vi "#24_MAV_MSG_GPS_RAW_INT.vi"(11 "mavlink_payload":u8[](array[numeric])) -> (3 "GPS_RAW_INT":T1)   [LabVIEW 2023]
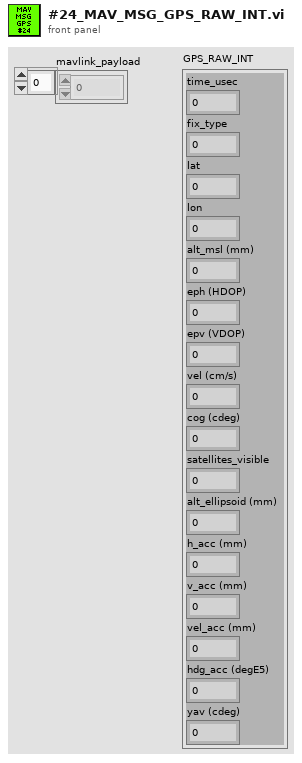
[diagram p1: front panel]
types:
  T1 = cluster{"time_usec":u64, "fix_type":u8, "lat":i32, "lon":i32, "alt_msl (mm)":i32, "eph (HDOP)":u16, "epv (VDOP)":u16, "vel (cm/s)":u16, "cog (cdeg)":u16, "satellites_visible":u8, "alt_ellipsoid (mm)":i32, "h_acc (mm)":u32, "v_acc (mm)":u32, "vel_acc (mm)":u32, "hdg_acc (degE5)":u32, "yav (cdeg)":u16}
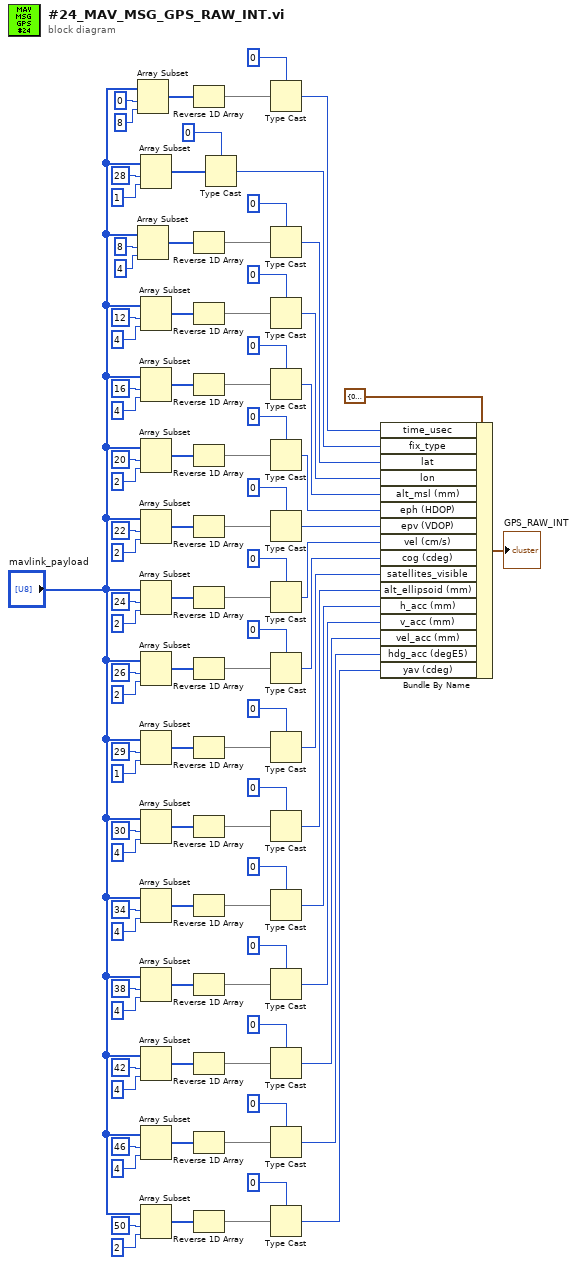
[diagram p0: block diagram]
diagram:
  n1 = Array Subset(array="mavlink_payload", index=0, length=8) -> (w98:u8[])
  n2 = Array Subset(array="mavlink_payload", index=8, length=4) -> (w82:u8[])
  n3 = Array Subset(array="mavlink_payload", index=28, length=1) -> (w88:u8[])
  n4 = Array Subset(array="mavlink_payload", index=12, length=4) -> (w76:u8[])
  n5 = Array Subset(array="mavlink_payload", index=16, length=4) -> (w70:u8[])
  n6 = Array Subset(array="mavlink_payload", index=20, length=2) -> (w65:u8[])
  n7 = Array Subset(array="mavlink_payload", index=22, length=2) -> (w59:u8[])
  n8 = Array Subset(array="mavlink_payload", index=24, length=2) -> (w53:u8[])
  n9 = Array Subset(array="mavlink_payload", index=26, length=2) -> (w47:u8[])
  n10 = Array Subset(array="mavlink_payload", index=29, length=1) -> (w41:u8[])
  n11 = Array Subset(array="mavlink_payload", index=30, length=4) -> (w35:u8[])
  n12 = Array Subset(array="mavlink_payload", index=34, length=4) -> (w29:u8[])
  n13 = Array Subset(array="mavlink_payload", index=38, length=4) -> (w23:u8[])
  n14 = Array Subset(array="mavlink_payload", index=42, length=4) -> (w17:u8[])
  n15 = Array Subset(array="mavlink_payload", index=46, length=4) -> (w11:u8[])
  n16 = Array Subset(array="mavlink_payload", index=50, length=2) -> (w5:u8[])
  n17 = Reverse 1D Array(array=w98) -> (reversed array=w97:u8[])
  n18 = Reverse 1D Array(array=w82) -> (reversed array=w81:u8[])
  n19 = Reverse 1D Array(array=w76) -> (reversed array=w75:u8[])
  n20 = Reverse 1D Array(array=w70) -> (reversed array=w69:u8[])
  n21 = Reverse 1D Array(array=w65) -> (reversed array=w64:u8[])
  n22 = Reverse 1D Array(array=w59) -> (reversed array=w58:u8[])
  n23 = Reverse 1D Array(array=w53) -> (reversed array=w52:u8[])
  n24 = Reverse 1D Array(array=w47) -> (reversed array=w46:u8[])
  n25 = Reverse 1D Array(array=w41) -> (reversed array=w40:u8[])
  n26 = Reverse 1D Array(array=w35) -> (reversed array=w34:u8[])
  n27 = Reverse 1D Array(array=w29) -> (reversed array=w28:u8[])
  n28 = Reverse 1D Array(array=w23) -> (reversed array=w22:u8[])
  n29 = Reverse 1D Array(array=w17) -> (reversed array=w16:u8[])
  n30 = Reverse 1D Array(array=w11) -> (reversed array=w10:u8[])
  n31 = Reverse 1D Array(array=w5) -> (reversed array=w4:u8[])
  n32 = Type Cast(type=u8 0 ("index"), x=w88) -> (*(type *) &x=w86:u8)
  n33 = Type Cast(type=u64 0 ("index"), x=w97) -> (*(type *) &x=w92:u64)
  n34 = Type Cast(type=0 ("index"), x=w81) -> (*(type *) &x=w80:i32)
  n35 = Type Cast(type=0 ("index"), x=w75) -> (*(type *) &x=w74:i32)
  n36 = Type Cast(type=0 ("index"), x=w69) -> (*(type *) &x=w56:i32)
  n37 = Type Cast(type=u16 0 ("index"), x=w64) -> (*(type *) &x=w63:u16)
  n38 = Type Cast(type=u16 0 ("index"), x=w58) -> (*(type *) &x=w57:u16)
  n39 = Type Cast(type=u16 0 ("index"), x=w52) -> (*(type *) &x=w50:u16)
  n40 = Type Cast(type=u16 0 ("index"), x=w46) -> (*(type *) &x=w44:u16)
  n41 = Type Cast(type=u8 0 ("index"), x=w40) -> (*(type *) &x=w38:u8)
  n42 = Type Cast(type=0 ("index"), x=w34) -> (*(type *) &x=w32:i32)
  n43 = Type Cast(type=u32 0 ("index"), x=w28) -> (*(type *) &x=w26:u32)
  n44 = Type Cast(type=u32 0 ("index"), x=w22) -> (*(type *) &x=w20:u32)
  n45 = Type Cast(type=u32 0 ("index"), x=w16) -> (*(type *) &x=w14:u32)
  n46 = Type Cast(type=u32 0 ("index"), x=w10) -> (*(type *) &x=w8:u32)
  n47 = Type Cast(type=u16 0 ("index"), x=w4) -> (*(type *) &x=w1:u16)
  n48 = Bundle By Name(cluster=T1 {"time_usec"=0, "fix_type"=0, "lat"=0, "lon"=0, "alt_msl (mm)"=0, "eph (HDOP)"=0, "epv (VDOP)"=0, "vel (cm/s)"=0, "cog (cdeg)"=0, "satellites_visible"=0, "alt_ellipsoid (mm)"=0, "h_acc (mm)"=0, "v_acc (mm)"=0, "vel_acc (mm)"=0, "hdg_acc (degE5)"=0, "yav (cdeg)"=0} ("GPS_RAW_INT"), "time_usec"=w92, "fix_type"=w86, "lat"=w80, "lon"=w74, "alt_msl (mm)"=w56, "eph (HDOP)"=w63, "epv (VDOP)"=w57, "vel (cm/s)"=w50, "cog (cdeg)"=w44, "satellites_visible"=w38, "alt_ellipsoid (mm)"=w32, "h_acc (mm)"=w26, "v_acc (mm)"=w20, "vel_acc (mm)"=w14, "hdg_acc (degE5)"=w8, "yav (cdeg)"=w1) -> (→"GPS_RAW_INT":T1)
